vi "AnalyzePortsHeader.vi"(0 "data":string) -> (1 "Input Names":string[](array[string]), 2 "Input Numbers":i32[](array[numeric]))   [LabVIEW 2010]
panel:
  out "array w/ subset deleted":string[](array[string])
  out "after substring":string
  out "array":string[][](array[string])
  out "subarray 2":string[](array[string])
  out "subarray":string[](array[string])
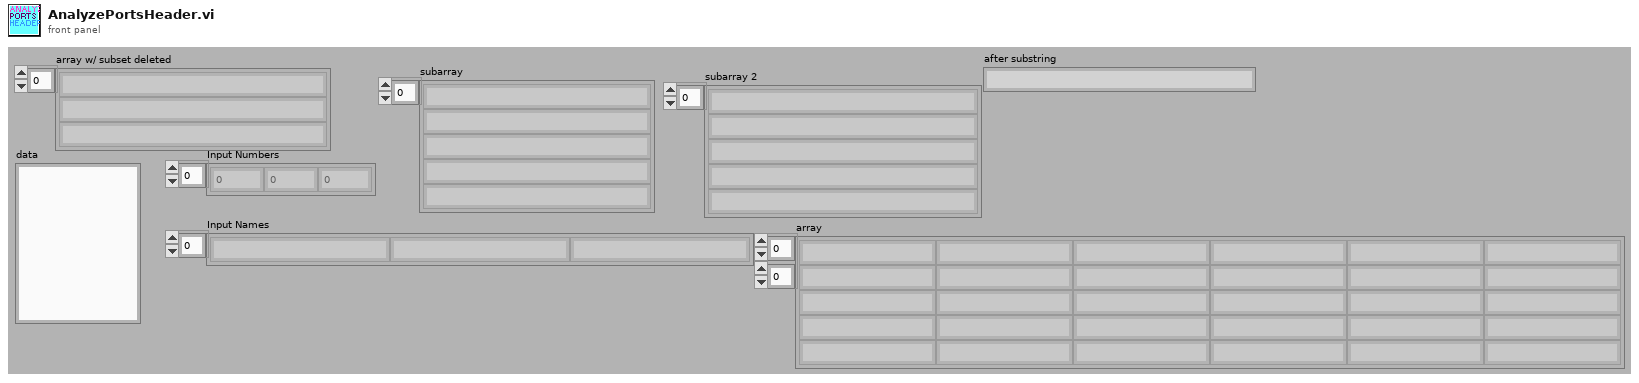
[diagram p1: front panel]
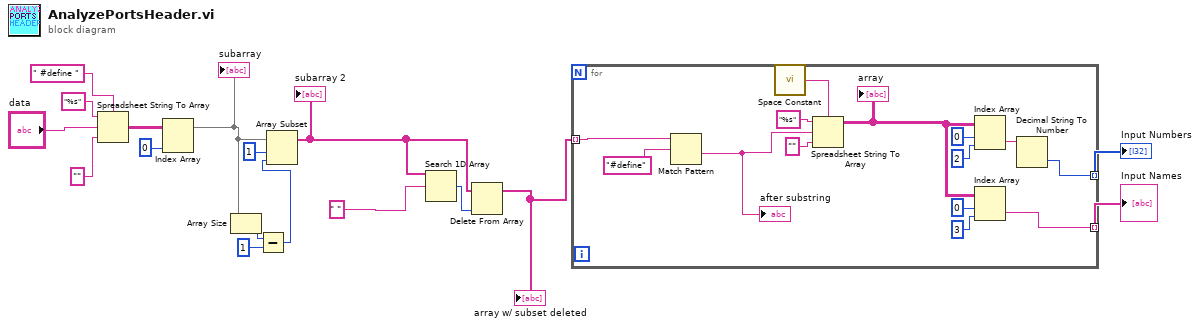
[diagram p0: block diagram]
diagram:
  n1 = Spreadsheet String To Array(delimiter (Tab)=" #define ", format string="%s", spreadsheet string="data", array type (2D Dbl)="" ("delimiter (Tab)")) -> (array=w9:string[][])
  n2 = Index Array(array=w9, index (col)=0 ("index (row)")) -> (element=w14:string[])  [unwired: 1 in]
  "subarray" <- w14
  n3 = Array Size(array=w14) -> (size(s)=w15:i32)
  n4 = Subtract(x=w15, y=1) -> (x-y=w16:i32)
  n5 = Array Subset(array=w14, index=1, length=w16) -> (w4:string[])
  "subarray 2" <- w4
  n6 = Search 1D Array(1D array=w4, element=" ") -> (index of element=w3:i32)  [unwired: 1 in]
  n7 = Delete From Array(array=w4, index=w3) -> (array with subset deleted=w1:string[])  [unwired: 1 in, 1 out]
  "array w/ subset deleted" <- w1
  n8 = for {
    tunnel: w1 -> [w21] mode=indexing
    tunnel: [w26] -> w12 mode=indexing
    tunnel: [w22] -> w13 mode=indexing
    n9 = Match Pattern(string=w21, regular expression="#define" ("delimiter (Tab)")) -> (after substring=w19:string)  [unwired: 1 in, 3 out]
    "after substring" <- w19
    n10 = call <vilib>:"Space Constant.vi"() -> ("String"=w18:string)
    n11 = Spreadsheet String To Array(delimiter (Tab)=w18, format string="%s", spreadsheet string=w19, array type (2D Dbl)="" ("delimiter (Tab)")) -> (array=w23:string[][])
    "array" <- w23
    n12 = Index Array(array=w23, index (row)=0, index (col)=2 ("disabled index (col)")) -> (element=w27:string)
    n13 = Index Array(array=w23, index (row)=0, index (col)=3 ("disabled index (col)")) -> (element=w22:string)
    n14 = Decimal String To Number(string=w27) -> (number=w26:i32)  [unwired: 2 in, 1 out]
  }
  "Input Numbers" <- w12
  "Input Names" <- w13
